vi "acquire.vi"() -> ()   [LabVIEW 2013]
uses:
  <vilib>/vision/NI_Vision_Development_Module.lvlib
panel:
  out "Reference Point in pixels\n (intersection)":cluster{"X":sgl, "Y":sgl} {"Y" format="%.2f"; "X" format="%.2f"}
  out "Circles Data (Circle Detection 1)":T1(array[cluster])
  out "Particle Measurements (Pixels) (Circle Analysis)":dbl[][](array[numeric]) format="%.2f"
  out "Number of Particles (Circle Analysis)":i32
  out "Image in":T2(plugin-control)
  in  "Stop":bool
  out "Binary":T2(plugin-control)
  in  "Capture image":bool
  out "Calibrated":T2(plugin-control)
  in  "File Path":path
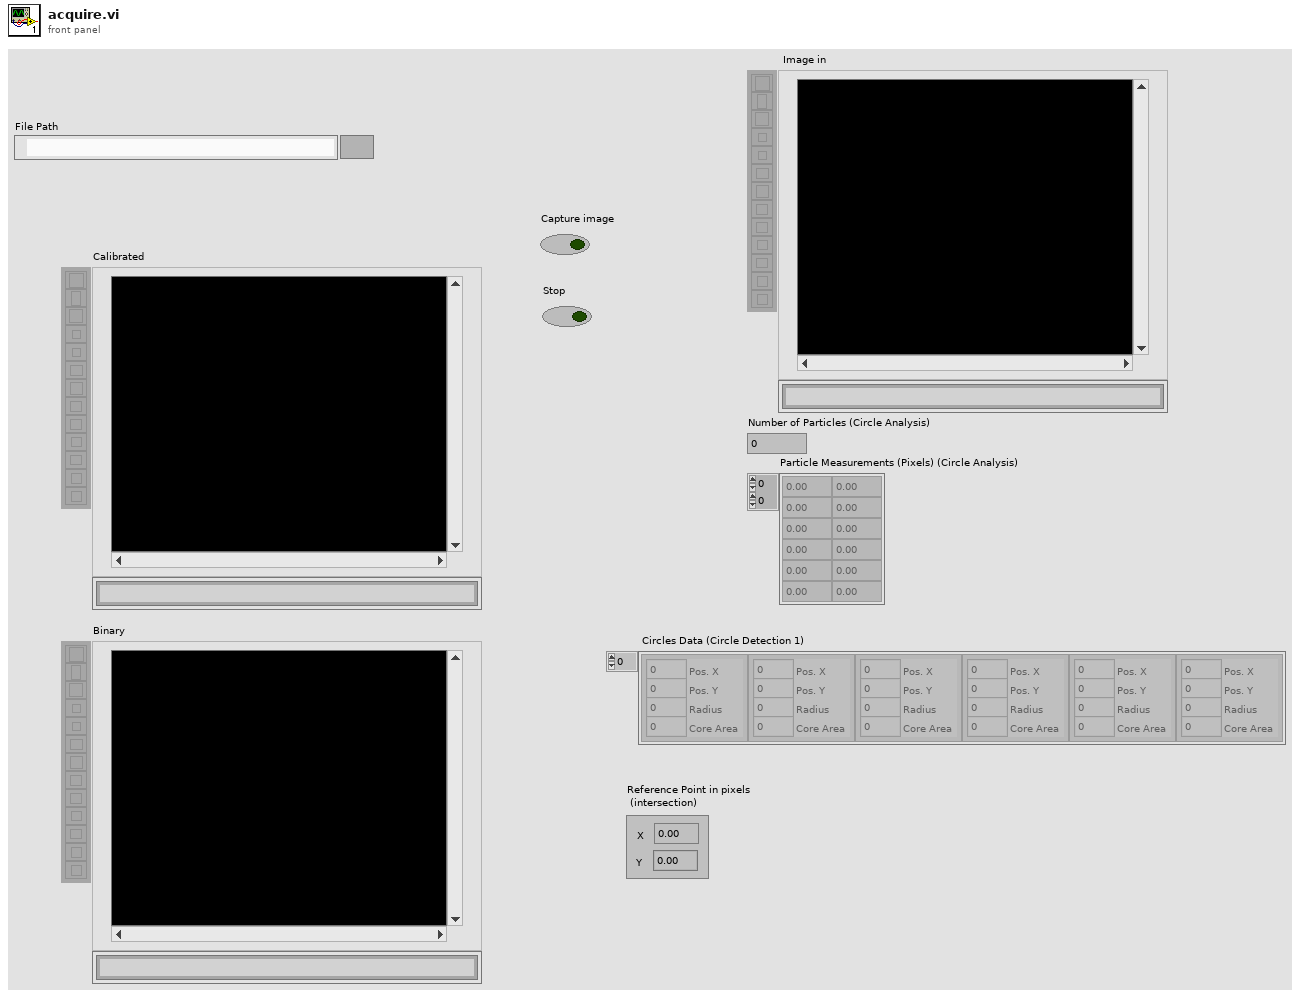
[diagram p1: front panel]
types:
  T1 = cluster{"Pos. X":i32, "Pos. Y":i32, "Radius":i32, "Core Area":i32}[]
  T2 = typedef "IMAQ Image.ctl" = refnum<image>
  T3 = typedef "Image Type" = u32
  T4 = cluster{"Point1 (Pixels)":cluster{"X":sgl, "Y":sgl}, "Point2 (Pixels)":cluster{"X":sgl, "Y":sgl}, "Point1 (Real-World)":cluster{"X":sgl, "Y":sgl}, "Point2 (Real-World)":cluster{"X":sgl, "Y":sgl}, "Angle (Pixel)":dbl, "Angle (Real-World)":dbl, "Score":dbl, "Straightness":dbl, "Average SNR (db)":dbl, "Calibration Valid":bool}
  T5 = cluster{"Point1 (Pixels)":cluster{"X":sgl, "Y":sgl}, "Point2 (Pixels)":cluster{"X":sgl, "Y":sgl}}
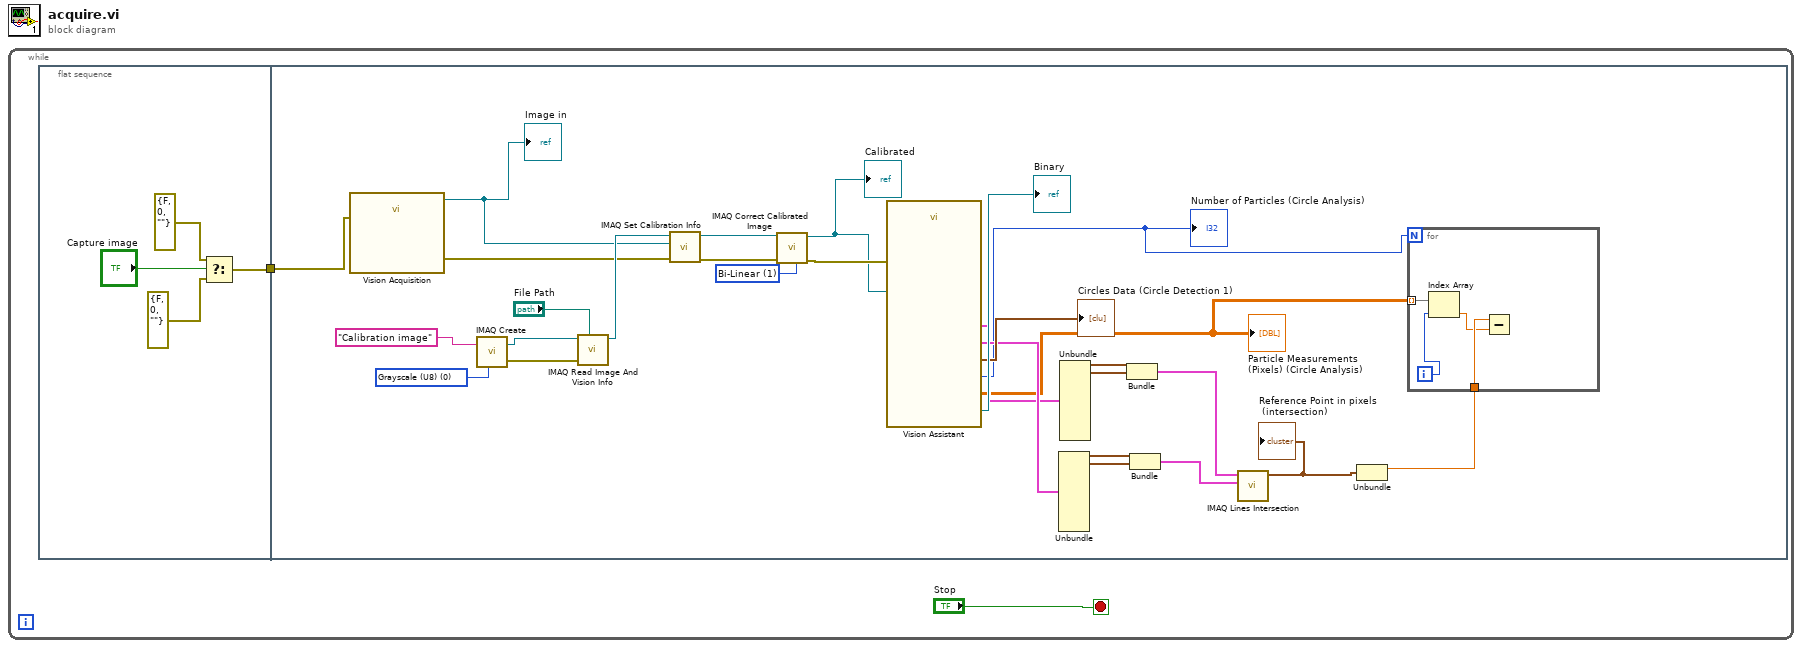
[diagram p0: block diagram]
diagram:
  n1 = while {
    stop <- "Stop" stop-if-true
    n2 = flat-sequence {
      tunnel: [w3] -> w1
      tunnel: w1 -> [w22]
      frame #0 {
        n3 = Select(t=errorcluster {"status"=FALSE, "code"=0, "source"=""} ("error in"), s="Capture image", f=errorcluster {"status"=FALSE, "code"=0, "source"=""} ("error in")) -> (s? t:f=w3:errorcluster)
      }
      frame #1 {
        w29 = T3 0 items=["Grayscale (U8)", "Grayscale (I16)", "Grayscale (SGL)", "Complex (CSG)", "RGB (U32)", "HSL (U32)", "RGB (U64)", "Grayscale (U16)"] ("Image Type")
        w28 = u32 1 items=["Zero Order", "Bi-Linear", "Quadratic", "Cubic Spline"] ("Interpolation Type")
        n4 = call "Vision Acquisition"("error in"=w22) -> ("Image Out"=w24:T2, "error out"=w23:errorcluster)  [unwired: 25 in]
        "Image in" <- w24
        n5 = call "IMAQ Create"("Image Name"="Calibration image", "Image Type"=w29) -> ("New Image"=w34:T2, "error out"=w33:errorcluster)  [unwired: 3 in]
        n6 = call "IMAQ Read Image And Vision Info"("File Path"="File Path", "error in (no error)"=w33, "Image"=w34) -> ("Image Out"=w32:T2)  [unwired: 6 in, 2 out]
        n7 = call "IMAQ Set Calibration Info"("error in (no error)"=w23, "Image Dst"=w24, "Image Src"=w32) -> ("error out"=w27:errorcluster, "Calibrated Image"=w31:T2)  [unwired: 7 in]
        n8 = call "IMAQ Correct Calibrated Image"("Interpolation Type"=w28, "error in (no error)"=w27, "Image Src"=w31) -> ("error out"=w26:errorcluster, "Corrected Image"=w19:T2)  [unwired: 7 in]
        "Calibrated" <- w19
        n9 = call "Vision Assistant"("Image In"=w19, "error in"=w26) -> ("Image Out"=→"Binary":T2, "Number of Particles (Circle Analysis)"=w9:i32, "Particle Measurements (Pixels) (Circle Analysis)"=w8:dbl[][], "Circles Data (Circle Detection 1)"=→"Circles Data (Circle Detection 1)":T1, "Straight Edge (Find Straight Edge 1)"=w14:T4, "Straight Edge (Find Straight Edge 2)"=w18:T4)  [unwired: 19 in, 1 out]
        "Number of Particles (Circle Analysis)" <- w9
        "Particle Measurements (Pixels) (Circle Analysis)" <- w8
        n10 = Unbundle(w18) -> ("Point1 (Pixels)"=w17:cluster{"X":sgl, "Y":sgl}, "Point2 (Pixels)"=w16:cluster{"X":sgl, "Y":sgl})  [unwired: 8 out]
        n11 = Unbundle(w14) -> ("Point1 (Pixels)"=w13:cluster{"X":sgl, "Y":sgl}, "Point2 (Pixels)"=w12:cluster{"X":sgl, "Y":sgl})  [unwired: 8 out]
        n12 = Bundle("Point1 (Pixels)"=w13, "Point2 (Pixels)"=w12) -> (w11:T5)  [unwired: 1 in]
        n13 = Bundle("Point1 (Pixels)"=w17, "Point2 (Pixels)"=w16) -> (w15:T5)  [unwired: 1 in]
        n14 = call "IMAQ Lines Intersection"("Line 2"=w15, "Line 1"=w11) -> ("Intersection Point"=w10:cluster{"X":sgl, "Y":sgl})  [unwired: 7 in, 2 out]
        "Reference Point in pixels\n (intersection)" <- w10
        n15 = Unbundle(w10) -> ("X"=w7:sgl)  [unwired: 1 out]
        n16 = for {
          N: w9 -> [_]
          tunnel: w8 -> [w37] mode=indexing
          tunnel: w7 -> [w36]
          i -> [w38]
          n17 = Index Array(array=w37, index=w38) -> (element=w35:dbl)
          n18 = Subtract(x=w36, y=w35) -> ()  [unwired: 1 out]
        }
      }
    }
  }
